vi "Movement_Control.vi"() -> ()   [LabVIEW 2017]
uses:
  <vilib>/myRIO/Instrument Drivers/Utilities/Utilities.lvlib
panel:
  in  "error in\n(no error)":errorcluster
  out "error out":errorcluster
  out "Battery Voltage \nOutput":u16
  in  "Omega":dbl
  in  "Vy":dbl
  in  "Vx":dbl
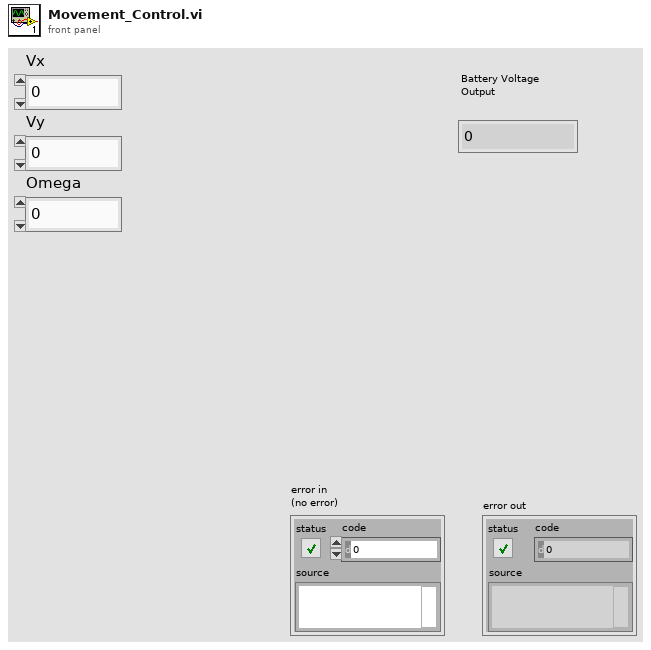
[diagram p1: front panel]
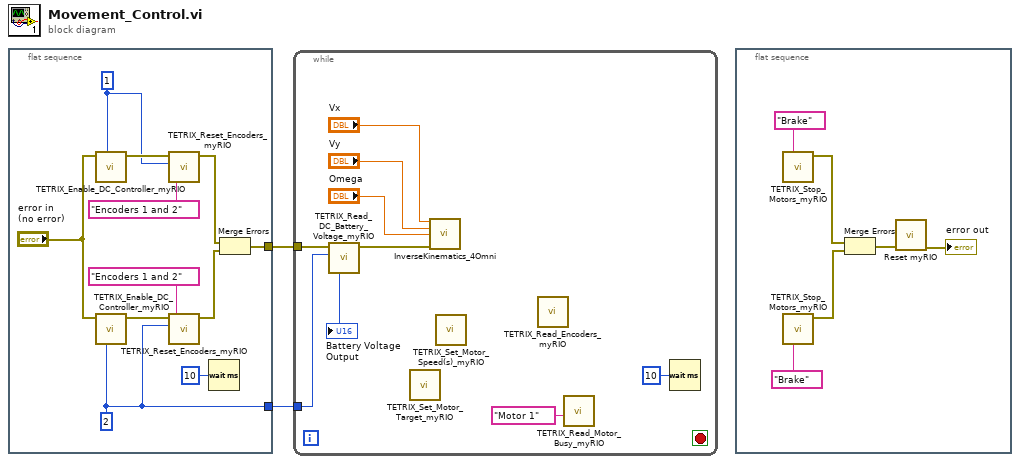
[diagram p0: block diagram]
diagram:
  n1 = flat-sequence {
    tunnel: [w6] -> w2
    tunnel: [w4] -> w1
    frame #0 {
      w11 = u8 1 ("Controller ID#  (I2C Address)")
      w4 = u8 2 ("Controller ID#  (I2C Address)")
      n2 = call <vilib>:"TETRIX_Enable_DC_Controller_myRIO.vi"("Controller ID#  (I2C Address)"=w11, "Error/Flow In"="error in\n(no error)") -> ("Error/Flow Out"=w12:errorcluster)  [unwired: 5 in]
      n3 = call <vilib>:"TETRIX_Enable_DC_Controller_myRIO.vi"("Controller ID#  (I2C Address)"=w4, "Error/Flow In"="error in\n(no error)") -> ("Error/Flow Out"=w13:errorcluster)  [unwired: 5 in]
      n4 = call <vilib>:"TETRIX_Reset_Encoders_myRIO.vi"("Select Encoder"="Encoders 1 and 2", "Controller ID#  (I2C Address)"=w11, "Error/Flow In"=w12) -> ("Error/Flow Out"=w8:errorcluster)  [unwired: 4 in]
      n5 = call <vilib>:"TETRIX_Reset_Encoders_myRIO.vi"("Select Encoder"="Encoders 1 and 2", "Controller ID#  (I2C Address)"=w4, "Error/Flow In"=w13) -> ("Error/Flow Out"=w7:errorcluster)  [unwired: 4 in]
      n6 = Wait (ms)(milliseconds to wait=u32 10) -> ()  [unwired: 1 out]
      n7 = Merge Errors(w8, w7) -> (w6:errorcluster)
    }
  }
  n8 = while {
    tunnel: w2 -> [w19]
    tunnel: w1 -> [w17]
    stop <- _ stop-if-true
    n9 = call <vilib>:"TETRIX_Read_DC_Battery_Voltage_myRIO.vi"("Controller ID#  (I2C Address)"=w17, "Error/Flow In"=w19) -> ("Error/Flow Out"=w18:errorcluster, "Battery Voltage Output"=→"Battery Voltage \nOutput":u16)  [unwired: 4 in]
    n10 = call <vilib>:"TETRIX_Set_Motor_Target_myRIO.vi"() -> ()  [unwired: 7 in, 1 out]
    n11 = call "InverseKinematics_4Omni.vi"("Vx"="Vx", "Vy"="Vy", "Omega"="Omega", "error in (no error)"=w18) -> ()  [unwired: 7 in, 5 out]
    n12 = call <vilib>:"TETRIX_Set_Motor_Speed(s)_myRIO.vi"() -> ()  [unwired: 7 in, 1 out]
    n13 = call <vilib>:"TETRIX_Read_Encoders_myRIO.vi"() -> ()  [unwired: 6 in, 2 out]
    n14 = call <vilib>:"TETRIX_Read_Motor_Busy_myRIO.vi"("Select Channel"="Motor 1") -> ()  [unwired: 5 in, 2 out]
    n15 = Wait (ms)(milliseconds to wait=u32 10) -> ()  [unwired: 1 out]
  }
  n16 = flat-sequence {
    frame #0 {
      n17 = call <vilib>:"TETRIX_Stop_Motors_myRIO.vi"("Stop Mode"="Brake") -> ("Error/Flow Out"=w28:errorcluster)  [unwired: 6 in]
      n18 = call <vilib>:"TETRIX_Stop_Motors_myRIO.vi"("Stop Mode"="Brake") -> ("Error/Flow Out"=w27:errorcluster)  [unwired: 6 in]
      n19 = Merge Errors(w28, w27) -> (w26:errorcluster)
      n20 = call <vilib>:"Reset myRIO.vi"("error in (no error)"=w26) -> ("error out"=→"error out":errorcluster)  [unwired: 10 in]
    }
  }
